vi "Color Sensor V3 CIE Lab Fcn.vi"(11 "x":dbl) -> (3 "y":dbl)   [LabVIEW 2019]
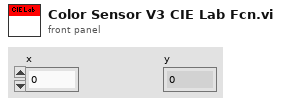
[diagram p1: front panel]
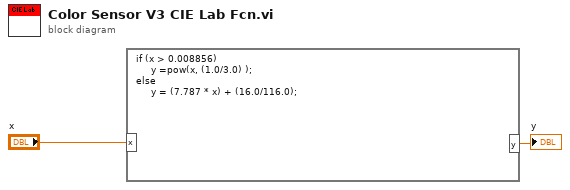
[diagram p0: block diagram]
diagram:
  n1 = formula code="if (x > 0.008856)\n     y =pow(x, (1.0/3.0) );\nelse\n     y = (7.787 * x) + (16.0/116.0);"("x"="x") -> ("y"=→"y":dbl)
